vi "GetPixelCalibrationHistogramReports.vi"(11 "Pixel calibration":T1) -> (2 "Gain Histogram Report":T3 {"Standard  Variation" format="%.2f"; "Mean Value" format="%.2f"; "Interval Width" format="%.2f"; "Starting Value" format="%.2f"; "Maximal Value" format="%.2f"; "Minimal Value" format="%.2f"}, 3 "Offset Histogram Report":T3 {"Standard  Variation" format="%.2f"; "Mean Value" format="%.2f"; "Interval Width" format="%.2f"; "Starting Value" format="%.2f"; "Maximal Value" format="%.2f"; "Minimal Value" format="%.2f"})   [LabVIEW 2011]
uses:
  PixelCalibrationDataType.ctl
  <vilib>/vision/Image Controls.llb/IMAQ Image.ctl
  <vilib>/vision/NI_Vision_Development_Module.lvlib
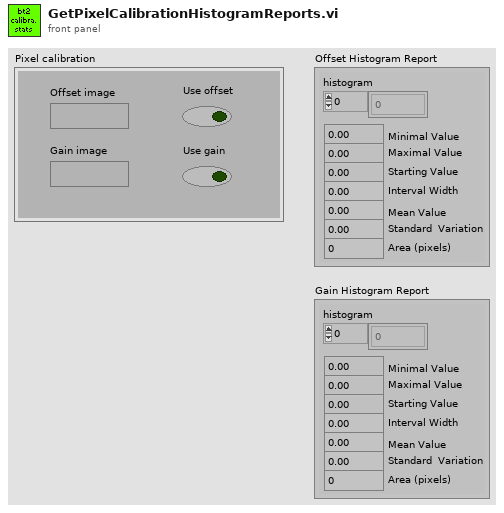
[diagram p1: front panel]
types:
  T1 = typedef "PixelCalibrationDataType.ctl" = cluster{"Offset image":T2, "Gain image":T2, "Use offset":bool, "Use gain":bool}
  T2 = typedef "IMAQ Image.ctl" = refnum<image>
  T3 = cluster{"histogram":u32[], "Minimal Value":sgl, "Maximal Value":sgl, "Starting Value":sgl, "Interval Width":sgl, "Mean Value":sgl, "Standard  Variation":sgl, "Area (pixels)":i32}
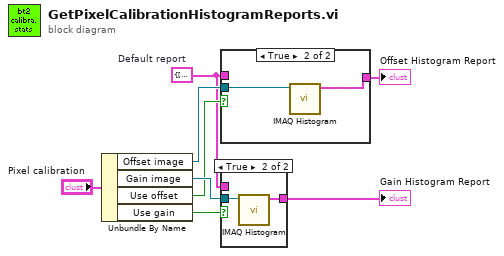
[diagram p0: block diagram]
diagram:
  w1 = T3 {"histogram"=[], "Minimal Value"=0.0, "Maximal Value"=0.0, "Starting Value"=0.0, "Interval Width"=0.0, "Mean Value"=0.0, "Standard  Variation"=0.0, "Area (pixels)"=0}  # Default report
  n1 = Unbundle By Name("Pixel calibration") -> ("Offset image"=w6:T2, "Gain image"=w5:T2, "Use offset"=w3:bool, "Use gain"=w4:bool)
  n2 = case shown="True" w3 {
    tunnel: w6 -> [_ w11]
    tunnel: [w9 w10] -> w7
    tunnel: w1 -> [w9 _]
    frame False {
    }
    frame True {
      n3 = call "IMAQ Histogram"("Image"=w11) -> ("Histogram Report"=w10:T3)  [unwired: 9 in, 1 out]
    }
  }
  "Offset Histogram Report" <- w7
  n4 = case shown="True" w4 {
    tunnel: w5 -> [_ w14]
    tunnel: [w12 w13] -> w8
    tunnel: w1 -> [w12 _]
    frame False {
    }
    frame True {
      n5 = call "IMAQ Histogram"("Image"=w14) -> ("Histogram Report"=w13:T3)  [unwired: 9 in, 1 out]
    }
  }
  "Gain Histogram Report" <- w8
